vi "Connect_PSU_GCFS.vi"(3 "error in (no error)":errorcluster, 5 "?":T1 {"Data Out Cluster"."Particle Measurements (Pixels) (Particle Analysis 1)" format="%.2f"}) -> (0 "error out":errorcluster, 1 "State out":string, 2 "output cluster":T1={"Core"={"Current VI Reference"=refnum, "Close Panel on Exit?"=FALSE}, "Your Boolean data"=FALSE, "Your string data"="", "Camera Cluster"={"Session"="", "Image"=refnum, "Position Image"=refnum, "PixelVal Image"=refnum, "Position Image Binary"=refnum, "Lable Image"=refnum}, "Data In Cluster"={"Images"={"Position Image path"=path "", "Sample folder path"=path "", "Label Image path"=path ""}, "Sample Name"="", "Sample Rate"=20, "Gradient Buffer"=0, "Data Acquisition.Setup.TempGrad"=0.0, "Control.PID gains"={"proportional gain (Kc)"=0.0, "integral time (Ti, min)"=0.0, "derivative time (Td, min)"=0.0}}, "Active"=FALSE, "Ready"=FALSE, "Exit"=FALSE, "Arduino"={"Connection"=FALSE, "Port"="", "State"=""}, "Program_Start"="", "Data Out Cluster"={"Particle Measurements (Pixels) (Particle Analysis 1)"=[], "Number of droplets"=0, "PosImg_Timestamp"=""}, "PSU"={"Connection"=FALSE, "Port"="", "State"=""}} {"Data Out Cluster"."Particle Measurements (Pixels) (Particle Analysis 1)" format="%.2f"})   [LabVIEW 2024]
uses:
  DataCluster_GCFS.ctl
  <vilib>/userDefined/High Color/IMAQdx.ctl
  <vilib>/vision/Image Controls.llb/IMAQ Image.ctl
  3fecfa67-3b21-477e-abb9-e6c266c22bf3.vi
  f28ec6ae-94ae-46b8-8c3f-28958ce1d9fa.vi
  a9b37c8b-7b1a-4864-ae66-bc56c044b39d.vi
  <vilib>/regexp/Match Regular Expression.xnode
panel:
  out "find list":string[](array[string])
  out "Connected?":bool
  out "Interface Description":string
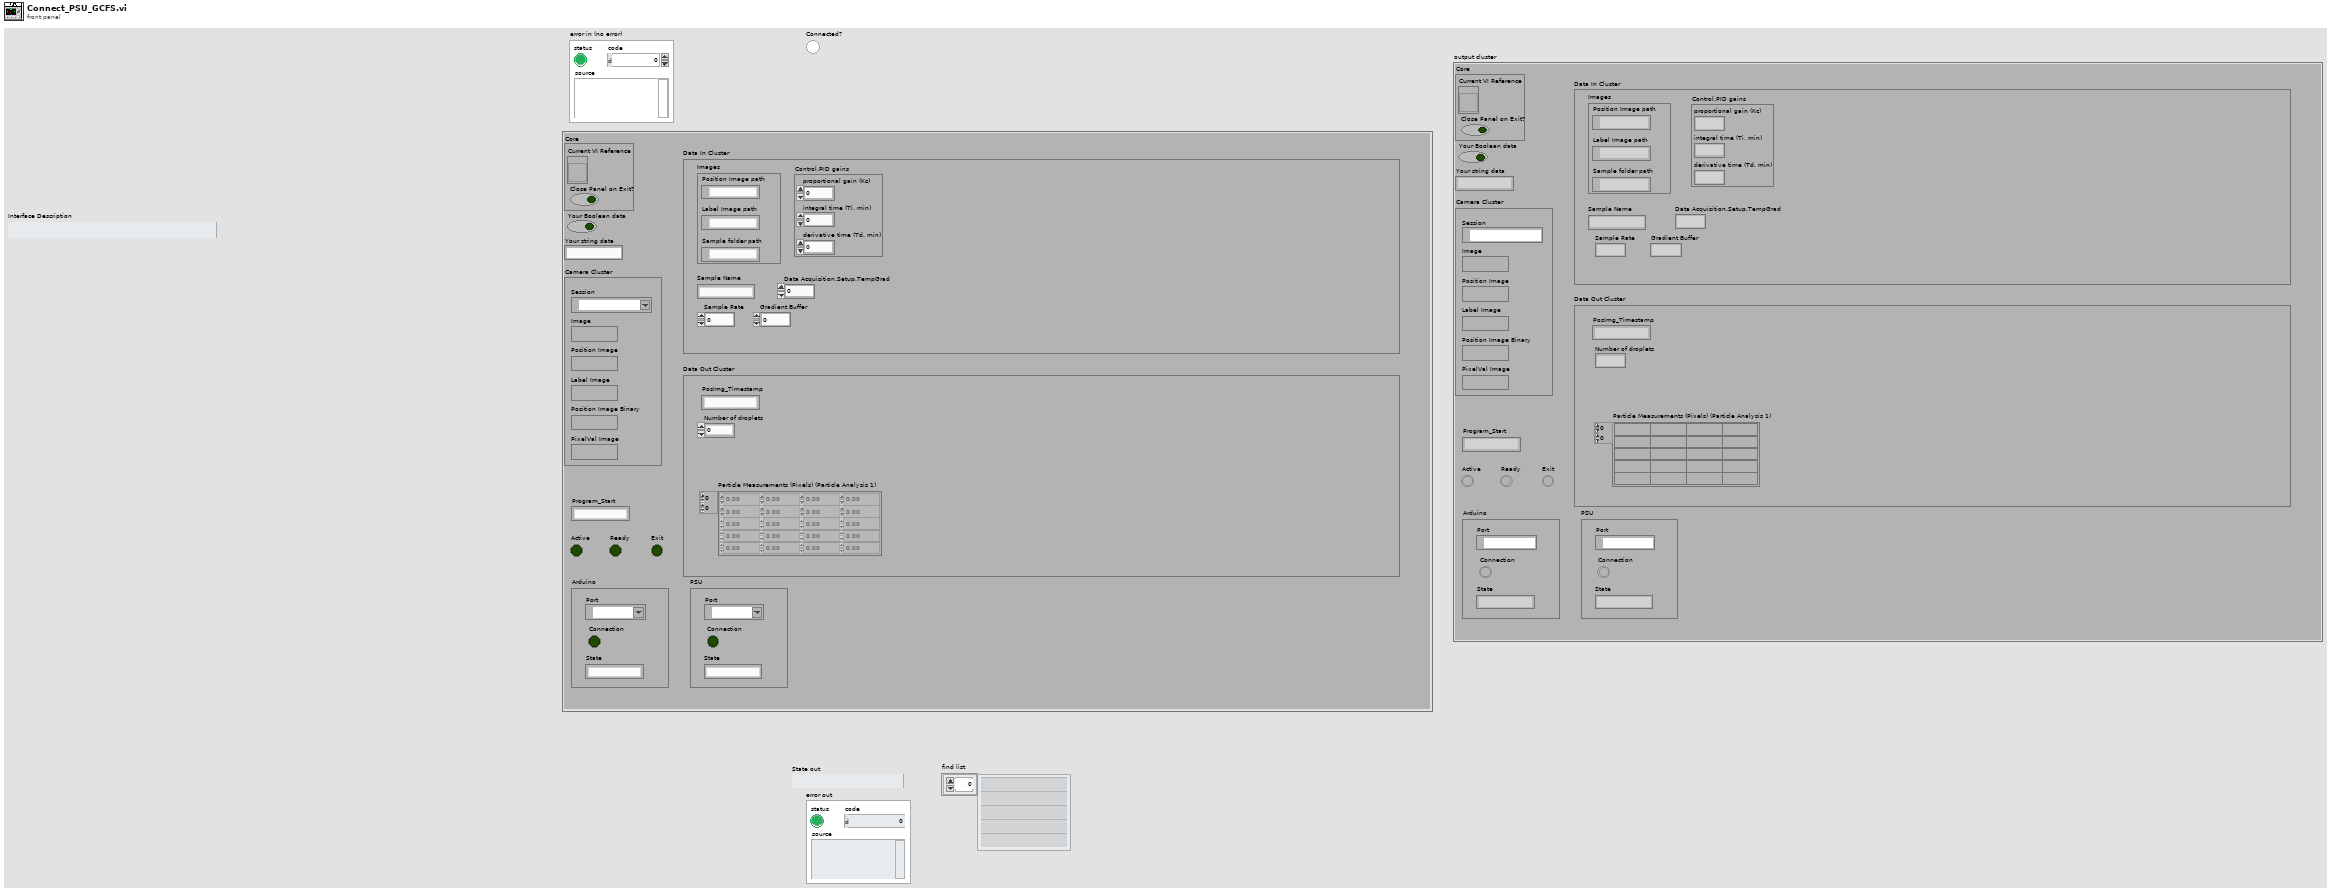
[diagram p1: front panel]
types:
  T1 = typedef "DataCluster_GCFS.ctl" = cluster{"Core":cluster{"Current VI Reference":refnum<vi>, "Close Panel on Exit?":bool}, "Your Boolean data":bool, "Your string data":string, "Camera Cluster":cluster{"Session":T2, "Image":T3, "Position Image":T3, "PixelVal Image":T3, "Position Image Binary":T3, "Lable Image":T3}, "Data In Cluster":cluster{"Images":cluster{"Position Image path":path, "Sample folder path":path, "Label Image path":path}, "Sample Name":string, "Sample Rate":i32, "Gradient Buffer":i32, "Data Acquisition.Setup.TempGrad":dbl, "Control.PID gains":cluster{"proportional gain (Kc)":dbl, "integral time (Ti, min)":dbl, "derivative time (Td, min)":dbl}}, "Active":bool, "Ready":bool, "Exit":bool, "Arduino":cluster{"Connection":bool, "Port":refnum<visa-resource-name>, "State":string}, "Program_Start":string, "Data Out Cluster":cluster{"Particle Measurements (Pixels) (Particle Analysis 1)":dbl[][], "Number of droplets":i32, "PosImg_Timestamp":string}, "PSU":cluster{"Connection":bool, "Port":refnum<visa-resource-name>, "State":string}}
  T2 = typedef "IMAQdx.ctl" = refnum<k21>
  T3 = typedef "IMAQ Image.ctl" = refnum<image>
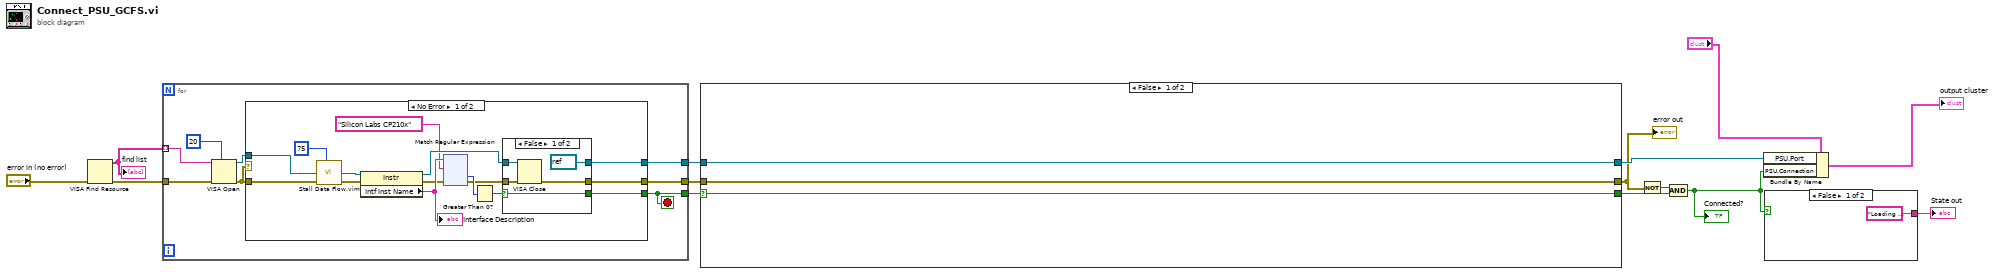
[diagram p0: block diagram]
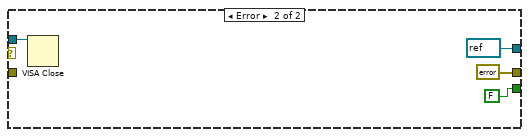
[diagram p4: hidden frame]
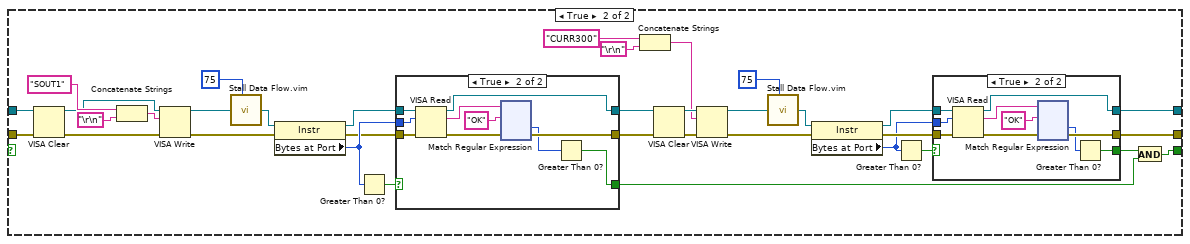
[diagram p5: hidden frame]
diagram:
  n1 = VISA Find Resource(8:"error in (no error)") -> (0:w13:errorcluster, 3:w14:string[])  [unwired: 2 in, 1 out]
  "find list" <- w14
  n2 = for {
    tunnel: w14 -> [w22] mode=indexing
    tunnel: w13 -> [w21]
    tunnel: [w18] -> w9
    tunnel: [w17] -> w11
    tunnel: [w19] -> w10
    stop <- w17 stop-if-true
    n3 = VISA Open(timeout (0)=u32 20 ("VISA Open timeout (0)"), error in (no error)=w21, VISA resource name=w22) -> (VISA resource name=w16:refnum<visa-resource-name>, error out=w20:errorcluster)  [unwired: 2 in]
    n4 = case shown="No Error" w20 {
      tunnel: w16 -> [w25 w163]
      tunnel: w20 -> [w36 _]
      tunnel: [w32 refnum<visa-resource-name> refnum ("Port")] -> w19
      tunnel: [w31 FALSE] -> w17
      tunnel: [w30 errorcluster {"status"=FALSE, "code"=0, "source"=""} ("error out")] -> w18
      frame No Error {
        n5 = call "Stall Data Flow.vim"("value in"=w25, "milliseconds to wait"=u32 75) -> ("value out"=w24:refnum<visa-resource-name>)  [unwired: 1 out]
        n6 = property class="Instr"(reference=w24, error in=w36) -> (reference out=w33:refnum<visa-resource-name>, error out=w27:errorcluster, "Intf Inst Name"=w35:string)
        "Interface Description" <- w35
        n7 = xnode "Match Regular Expression"("input string"=w35, "regular expression"="Silicon Labs CP210x", "error in"=w27) -> ("offset past match"=w28:i32, "error out"=w26:errorcluster)  [unwired: 3 in, 3 out]
        n8 = Greater Than 0?(x=w28) -> (x > 0?=w34:bool)
        n9 = case shown="False" w34 {
          selector: w34 -> [w158 w160]
          tunnel: w33 -> [w157 w161]
          tunnel: [refnum<visa-resource-name> refnum ("Port") w161] -> w32
          tunnel: [w158 w160] -> w31
          tunnel: w26 -> [w156 w159]
          tunnel: [w155 w159] -> w30
          frame False {
            n10 = VISA Close(VISA resource name=w157, error in (no error)=w156) -> (error out=w155:errorcluster)
          }
          frame True {
          }
        }
      }
      frame Error {
        n11 = VISA Close(VISA resource name=w163) -> ()  [unwired: 1 in, 1 out]
      }
    }
  }
  n12 = case shown="False" w11 {
    selector: w11 -> [w167 _]
    tunnel: w10 -> [w166 w200]
    tunnel: w9 -> [w168 w199]
    tunnel: [w166 w171] -> w8
    tunnel: [w168 w172] -> w5
    tunnel: [w167 w170] -> w7
    frame False {
    }
    frame True {
      n13 = VISA Clear(VISA resource name=w200, error in (no error)=w199) -> (VISA resource name out=w198:refnum<visa-resource-name>, error out=w197:errorcluster)
      n14 = Concatenate Strings("SOUT1" ("string"), "\r\n") -> (w201:string)
      n15 = VISA Write(VISA resource name=w198, write buffer=w201, error in (no error)=w197) -> (VISA resource name out=w190:refnum<visa-resource-name>, error out=w189:errorcluster)  [unwired: 1 out]
      n16 = call "Stall Data Flow.vim"("value in"=w190, "milliseconds to wait"=u32 75) -> ("value out"=w196:refnum<visa-resource-name>)  [unwired: 1 out]
      n17 = property class="Instr"(reference=w196, error in=w189) -> (reference out=w193:refnum<visa-resource-name>, error out=w192:errorcluster, "Bytes at Port"=w194:u32)
      n18 = Greater Than 0?(x=w194) -> (x > 0?=w195:bool)
      n19 = case shown="True" w195 {
        selector: w195 -> [w334 _]
        tunnel: w194 -> [_ w346]
        tunnel: w192 -> [w335 w345]
        tunnel: [w336 w344] -> w174
        tunnel: [w335 w339] -> w173
        tunnel: w193 -> [w336 w343]
        tunnel: [w334 w337] -> w188
        frame False {
        }
        frame True {
          n20 = VISA Read(VISA resource name=w343, byte count=w346, error in (no error)=w345) -> (VISA resource name out=w344:refnum<visa-resource-name>, read buffer=w342:string, error out=w341:errorcluster)  [unwired: 1 out]
          n21 = xnode "Match Regular Expression"("input string"=w342, "regular expression"="OK", "error in"=w341) -> ("offset past match"=w338:i32, "error out"=w339:errorcluster)  [unwired: 3 in, 3 out]
          n22 = Greater Than 0?(x=w338) -> (x > 0?=w337:bool)
        }
      }
      n23 = Concatenate Strings("CURR300" ("string"), "\r\n") -> (w178:string)
      n24 = VISA Clear(VISA resource name=w174, error in (no error)=w173) -> (VISA resource name out=w179:refnum<visa-resource-name>, error out=w180:errorcluster)
      n25 = VISA Write(VISA resource name=w179, write buffer=w178, error in (no error)=w180) -> (VISA resource name out=w186:refnum<visa-resource-name>, error out=w187:errorcluster)  [unwired: 1 out]
      n26 = call "Stall Data Flow.vim"("value in"=w186, "milliseconds to wait"=u32 75) -> ("value out"=w181:refnum<visa-resource-name>)  [unwired: 1 out]
      n27 = property class="Instr"(reference=w181, error in=w187) -> (reference out=w184:refnum<visa-resource-name>, error out=w185:errorcluster, "Bytes at Port"=w183:u32)
      n28 = Greater Than 0?(x=w183) -> (x > 0?=w182:bool)
      n29 = case shown="True" w182 {
        selector: w182 -> [w204 _]
        tunnel: w183 -> [_ w216]
        tunnel: w185 -> [w205 w215]
        tunnel: [w206 w214] -> w171
        tunnel: [w205 w209] -> w172
        tunnel: w184 -> [w206 w213]
        tunnel: [w204 w207] -> w169
        frame False {
        }
        frame True {
          n30 = VISA Read(VISA resource name=w213, byte count=w216, error in (no error)=w215) -> (VISA resource name out=w214:refnum<visa-resource-name>, read buffer=w212:string, error out=w211:errorcluster)  [unwired: 1 out]
          n31 = xnode "Match Regular Expression"("input string"=w212, "regular expression"="OK", "error in"=w211) -> ("offset past match"=w208:i32, "error out"=w209:errorcluster)  [unwired: 3 in, 3 out]
          n32 = Greater Than 0?(x=w208) -> (x > 0?=w207:bool)
        }
      }
      n33 = And(x=w169, y=w188) -> (x .and. y?=w170:bool)
    }
  }
  "error out" <- w5
  n34 = Not(x=w5) -> (.not. x?=w3:bool)
  n35 = And(x=w3, y=w7) -> (x .and. y?=w4:bool)
  "Connected?" <- w4
  n36 = Bundle By Name(cluster="?", "PSU.Port"=w8, "PSU.Connection"=w4) -> (→"output cluster":T1)
  n37 = case shown="False" w4 {
    tunnel: ["Loading UI: Description >> PSU Connection Failed!" _] -> w6
    frame False {
    }
    frame True {
    }
  }
  "State out" <- w6
